vi "Read Metadata.vi"(8 "error in (no error)":errorcluster, 10 "Plugin Info in":T1, 11 "metadata ref in":T5) -> (0 "error out":errorcluster, 2 "Plugin Info out":T1, 3 "metadata ref dup":T5)   [LabVIEW 2021, in "CIFPluginManager.lvclass"]
uses:
  CIFPluginManager.lvclass
  <vilib>/Utility/config.llb/Config Data RefNum.ctl
  typedef/Discovered Plugin.ctl
  CIFCore/Common/Typedef/Version.ctl
  typedef/Plugin Metadata.ctl
  typedef/Loader Type.ctl
  <vilib>/Utility/config.llb/Read Key (String).vi
  <vilib>/Utility/config.llb/NI_LVConfig.lvlib
  CIFCore/Common/CIFCoreCommon.lvlib
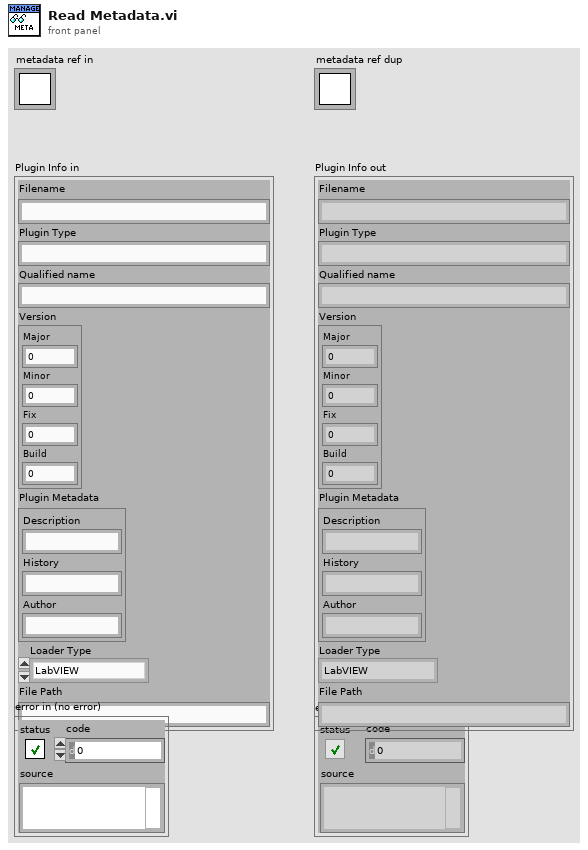
[diagram p1: front panel]
types:
  T1 = typedef "CIFPluginManager.lvclass/Discovered Plugin.ctl" = cluster{"Filename":string, "Plugin Type":string, "Qualified name":string, "Version":T2, "Plugin Metadata":T3, "Loader Type":T4, "File Path":string}
  T2 = typedef "CIFCoreCommon.lvlib/Version.ctl" = cluster{"Major":i32, "Minor":i32, "Fix":i32, "Build":i32}
  T3 = typedef "CIFPluginManager.lvclass/Plugin Metadata.ctl" = cluster{"Description":string, "History":string, "Author":string}
  T4 = typedef "CIFPluginManager.lvclass/Loader Type.ctl" = enum16{"LabVIEW"}
  T5 = typedef "NI_LVConfig.lvlib/Config Data RefNum.ctl" = refnum<k1>
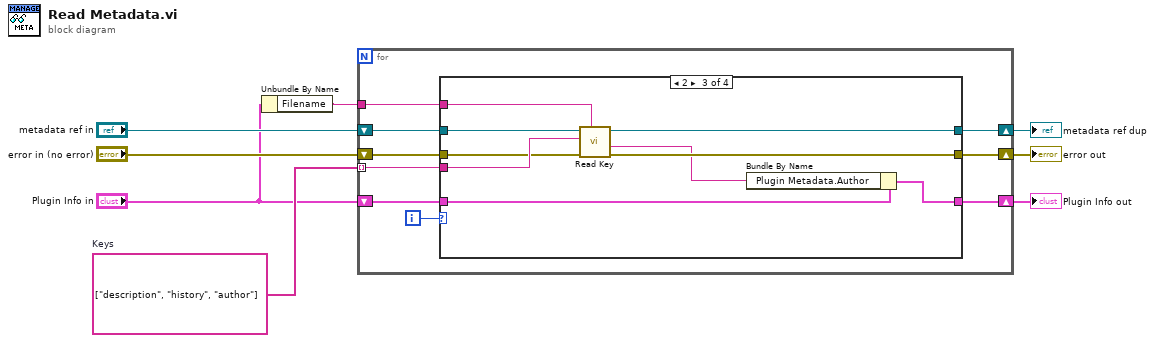
[diagram p0: block diagram]
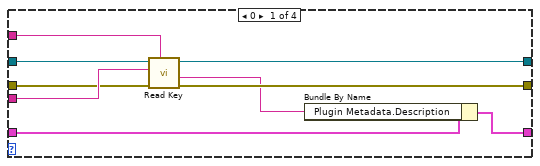
[diagram p2: hidden frame]
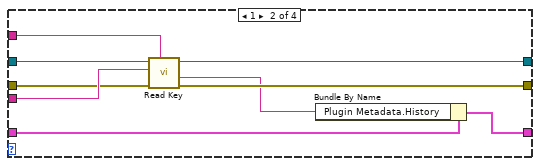
[diagram p3: hidden frame]
diagram:
  w6 = string[] ["description", "history", "author"]  # Keys
  n1 = Unbundle By Name("Plugin Info in") -> ("Filename"=w7:string)
  n2 = for {
    tunnel: w7 -> [w16]
    tunnel: w6 -> [w15] mode=indexing
    shift-right: [w13] -> w3
    shift-left: "error in (no error)" -> [w14]
    shift-right: [w12] -> w4
    shift-left: "metadata ref in" -> [w17]
    shift-right: [w9] -> w1
    shift-left: "Plugin Info in" -> [w10]
    i -> [w11]
    n3 = case shown="2" w11 {
      tunnel: w17 -> [w26 w35 w44 w47]
      tunnel: w16 -> [w25 w34 w43 _]
      tunnel: w15 -> [w24 w33 w42 _]
      tunnel: w14 -> [w23 w32 w41 w46]
      tunnel: [w22 w31 w40 w46] -> w13
      tunnel: [w21 w30 w39 w47] -> w12
      tunnel: w10 -> [w20 w29 w38 w45]
      tunnel: [w18 w27 w36 w45] -> w9
      frame 0 {
        n4 = call-poly <vilib>:"Read Key.vi"("section"=w25, "error in (no error)"=w23, "key"=w24, "refnum"=w26) -> ("error out"=w22:errorcluster, "value"=w19:string, "refnum out"=w21:T5)  [unwired: 4 in, 1 out]
        n5 = Bundle By Name(cluster=w20, "Plugin Metadata.Description"=w19) -> (w18:T1)
      }
      frame 1 {
        n6 = call-poly <vilib>:"Read Key.vi"("section"=w34, "error in (no error)"=w32, "key"=w33, "refnum"=w35) -> ("error out"=w31:errorcluster, "value"=w28:string, "refnum out"=w30:T5)  [unwired: 4 in, 1 out]
        n7 = Bundle By Name(cluster=w29, "Plugin Metadata.History"=w28) -> (w27:T1)
      }
      frame 2 {
        n8 = call-poly <vilib>:"Read Key.vi"("section"=w43, "error in (no error)"=w41, "key"=w42, "refnum"=w44) -> ("error out"=w40:errorcluster, "value"=w37:string, "refnum out"=w39:T5)  [unwired: 4 in, 1 out]
        n9 = Bundle By Name(cluster=w38, "Plugin Metadata.Author"=w37) -> (w36:T1)
      }
      frame -1, Default {
      }
    }
  }
  "metadata ref dup" <- w4
  "error out" <- w3
  "Plugin Info out" <- w1
